vi "UDP Data Link - Configuration Utilities - Set Time Stamp.vi"(8 "error in (no error)":errorcluster, 11 "Device Item Ref in":T1 format="%.0x") -> (0 "error out":errorcluster, 2 "Path":string, 3 "Device Item Ref out":T1 format="%.0x")   [LabVIEW 2012, in "UDP Data Link System Explorer.lvlib"]
doc: "Set the TimeStamp Ref Device Property to the System Time channel."
uses:
  UDP Data Link System Explorer.lvlib
  <vilib>/NI Veristand/Custom Device API/Custom Device Item Ref.ctl
  Shared/UDP Data Link Global.vi
  <vilib>/NI Veristand/Custom Device API/Set Item Property (Dependent Node Pointer).vi
  <vilib>/NI Veristand/Custom Device API/Custom Device API.lvlib
  <vilib>/NI Veristand/Custom Device Tools/Custom Device Utility Library/Custom Device Utility Library.lvlib
  Shared/UDP Data Link Shared.lvlib
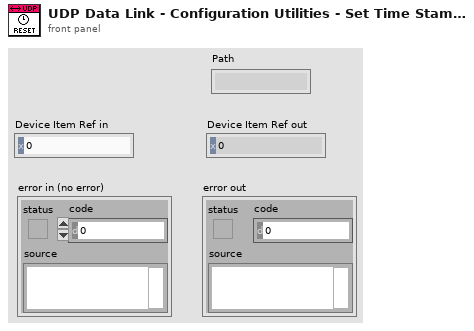
[diagram p1: front panel]
types:
  T1 = typedef "Custom Device API.lvlib/Custom Device Item Ref.ctl" = u64
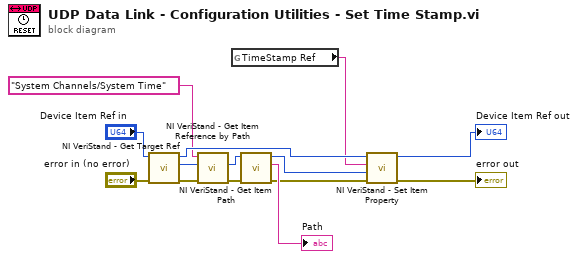
[diagram p0: block diagram]
diagram:
  n1 = call <vilib>:"NI VeriStand - Get Target Ref.vi"("error in"="error in (no error)", "Item Ref in"="Device Item Ref in") -> ("error out"=w13:errorcluster, "Target Ref"=w14:T1, "Item Ref out"=w12:T1)  [unwired: 6 in, 1 out]
  n2 = call <vilib>:"NI VeriStand - Get Item Reference by Path.vi"("error in (no error)"=w13, "Root Ref"=w14, "Item Path in"="System Channels/System Time" ("Relative Item Path")) -> ("error out"=w4:errorcluster, "Item Ref"=w5:T1)  [unwired: 5 in, 2 out]
  n3 = global read "UDP Data Link Global.vi" "TimeStamp Ref"() -> (w6:string)
  n4 = call <vilib>:"NI VeriStand - Get Item Path.vi"("error in (no error)"=w4, "Item Ref in"=w5) -> ("error out"=w1:errorcluster, "Path"=→"Path":string, "Item Ref out"=w2:T1)  [unwired: 6 in, 1 out]
  n5 = call-poly <vilib>:"NI VeriStand - Set Item Property.vi"("error in (no error)"=w1, "Dependent Node Ref"=w2, "Property Name"=w6, "Item Ref in"=w12) -> ("error out"=→"error out":errorcluster, "Item Ref out"=→"Device Item Ref out":T1)  [unwired: 5 in, 1 out]
